vi "Drive Published Globals.vi"() -> ()   [LabVIEW 2018]
doc: "This is used primarily to publish values that other subsystems or user code may want to read periodically. It may also contain some settings such as debug switches or implementation selections that are independent of the operating mode of the subsystem."
uses:
  Drive Setpoints.ctl
  Drive Operations.ctl
  Support Code/Path Data.ctl
  Support Code/Availible Command systems for auto.ctl
  <vilib>/Rock Robotics/WPI/Framework/Command Status Info.ctl
  <vilib>/Rock Robotics/WPI/Framework/Completion Status.ctl
  <vilib>/Rock Robotics/WPI/Framework/Completion Notifier.ctl
panel:
  out "Current Command":T8 {"SubSystem Data"."Auto Path Data"."Commands"."System" items=["FLoating Intake"=2, "Carriage Intake"=1, "Elevator"=0]; "SubSystem Data"."Auto Path Data"."Commands"."System Selection" items=["FLoating Intake"=2, "Carriage Intake"=1, "Elevator"=0]; "?"."SubSystem Data"."Auto Path Data"."Commands"."System" items=["FLoating Intake"=2, "Carriage Intake"=1, "Elevator"=0]; "?"."SubSystem Data"."Auto Path Data"."Commands"."System Selection" items=["FLoating Intake"=2, "Carriage Intake"=1, "Elevator"=0]}
  in  "Encoder Right":dbl
  in  "Encoder Left":dbl
  # "Tip: The global is a good way publish state or\ninformational/debugging values.\nIt is not  advised that you put setpoint values here."
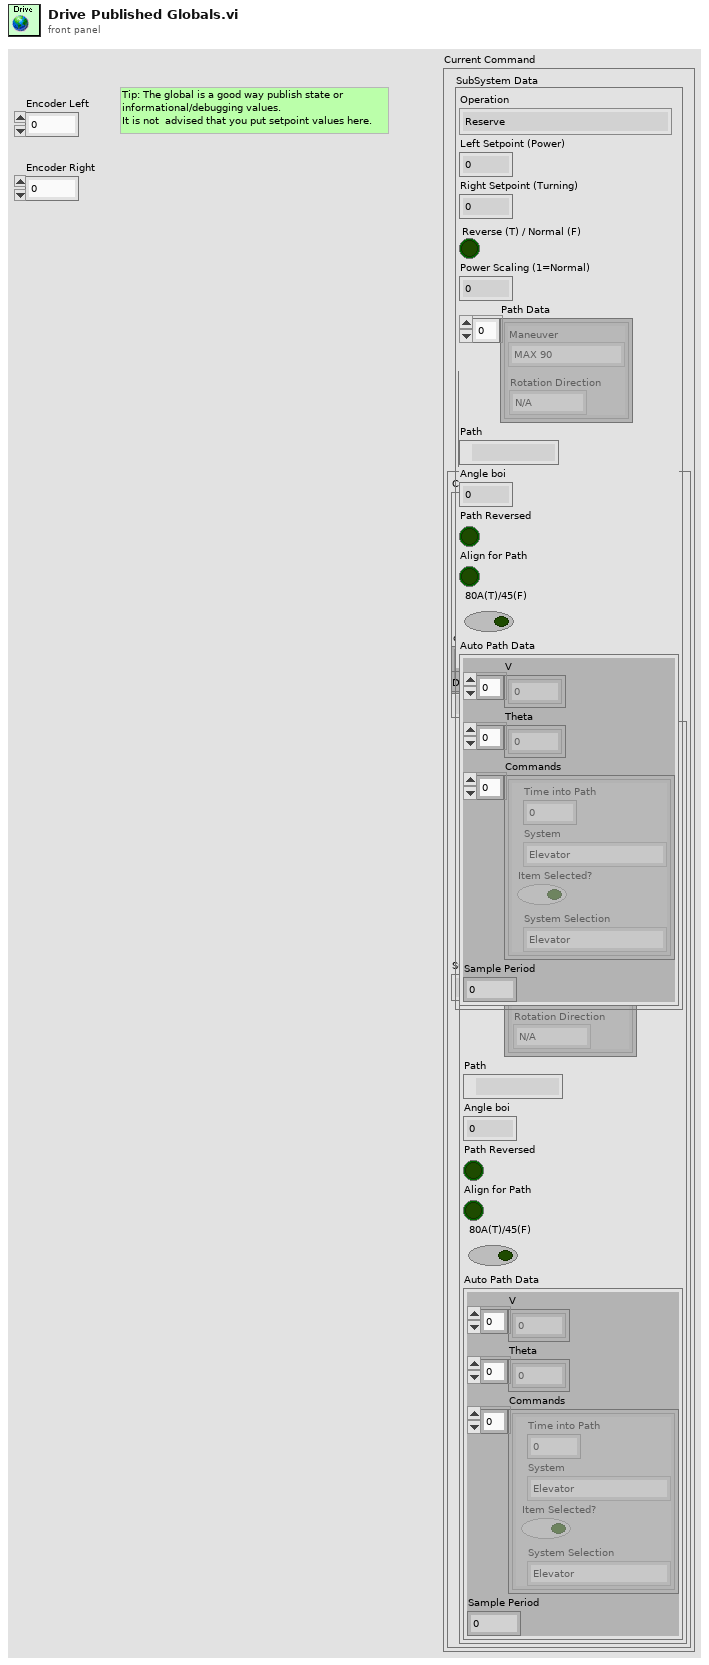
[diagram p1: front panel]
types:
  T1 = typedef "Drive Setpoints.ctl" = cluster{"Operation":T2, "Left Setpoint (Power)":dbl, "Right Setpoint (Turning)":dbl, "Reverse (T) / Normal (F)":bool, "Power Scaling (1=Normal) ":dbl, "Path Data":T3, "Path":path, "Angle boi":dbl, "Path Reversed":bool, "Align for Path":bool, "80A(T)/45(F)":bool, "Auto Path Data":cluster{"V":dbl[], "Theta":dbl[], "Commands":cluster{"Time into Path":dbl, "System":T4, "Item Selected?":bool, "System Selection":T4}[], "Sample Period":dbl}}
  T2 = typedef "Drive Operations.ctl" = enum16{"Reserve", "Read Current", "Immediate", "J-Turn", "Play Back From Log", "Auto-Align"}
  T3 = typedef "Path Data.ctl" = cluster{"Maneuver":enum16{"MAX 90", "MAX 180", "Turn to Home", "Turn to Rocket", "Auto-Align", "Turn to ..."}, "Rotation Direction":enum16{"N/A", "Right", "Left"}}[]
  T4 = typedef "Availible Command systems for auto.ctl" = u16
  T5 = typedef "Command Status Info.ctl" = cluster{"Name":string, "Status":T6, "notifier out":T7}
  T6 = typedef "Completion Status.ctl" = enum16{"Successful", "Aborted", "Incomplete"}
  T7 = typedef "Completion Notifier.ctl" = refnum<notifier>
  T8 = cluster{"SubSystem Data":T1, cluster{"Start Time (ms)":u32, "Iterations":i32}, cluster{"Command Info":T5, "Description":string, "SubSystem Data":T1, "queue out":refnum<queue>, "Subsystem Name":string}}
diagram:
